vi "id.To JSON Tree.vi"(8 "error in (no error)":errorcluster, 11 "id in":refnum<class "id.lvclass">) -> (0 "error out":errorcluster, 2 "JSON Value out":variant, 3 "id out":refnum<class "id.lvclass">)   [LabVIEW 2020, in "JSON-RPC Lib.lvlib" / "id.lvclass"]
uses:
  id.lvclass
  id.lvclass/id.ctl
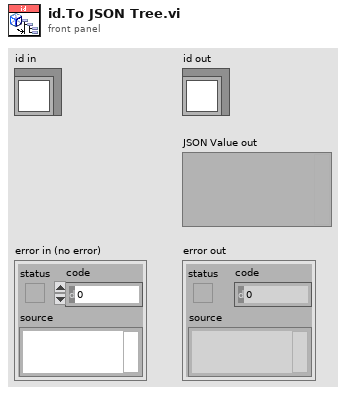
[diagram p1: front panel]
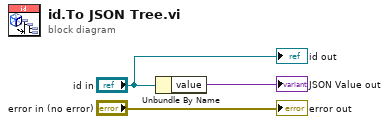
[diagram p0: block diagram]
diagram:
  n1 = Unbundle By Name("id in") -> ("value"=→"JSON Value out":variant)
  "error out" <- "error in (no error)"
  "id out" <- "id in"
